vi "Read handler properties.vi"(11 "basic HTTP handler dataset in":refnum<class "HTTPS handler dataset.lvclass">) -> (2 "server properties":T1={"max url size"=8000, "max header"=8000, "timeout ms"=5000, "max data size"=104857600}, 3 "basic HTTP handler dataset out":refnum<class "HTTPS handler dataset.lvclass">)   [LabVIEW 2016, in "HTTPS handler dataset.lvclass"]
uses:
  HTTPS handler dataset.lvclass
  HTTP server/http server properties.ctl
  HTTPS handler dataset.lvclass/HTTPS handler dataset.ctl
  HTTP server/Basic HTTPS server.lvclass
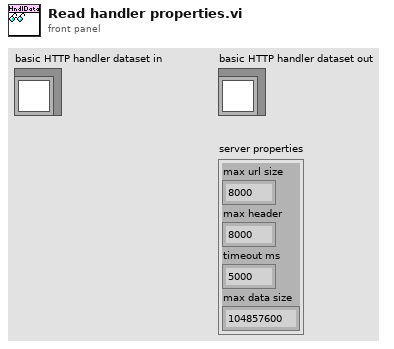
[diagram p1: front panel]
types:
  T1 = typedef "Basic HTTPS server.lvclass/http server properties.ctl" = cluster{"max url size":i32, "max header":i32, "timeout ms":i32, "max data size":i32}
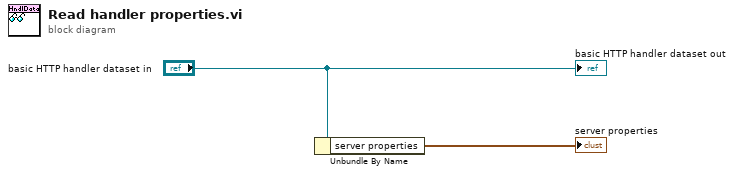
[diagram p0: block diagram]
diagram:
  n1 = Unbundle By Name("basic HTTP handler dataset in") -> ("server properties"=→"server properties":T1)
  "basic HTTP handler dataset out" <- "basic HTTP handler dataset in"
